vi "End.vi"(8 "error in (no error)":errorcluster, 11 "TelFocus in":refnum<class "TelFocus.lvclass">) -> (0 "error out":errorcluster, 3 "TelFocus out":refnum<class "TelFocus.lvclass">)   [LabVIEW 2018, in "TelFocus.lvclass"]
uses:
  TelFocus.lvclass
  Server/Server.lvclass
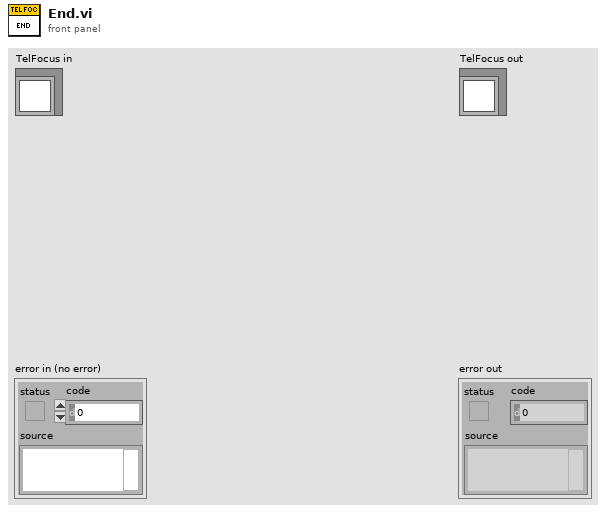
[diagram p1: front panel]
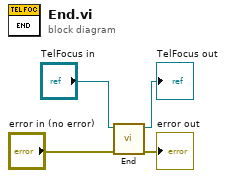
[diagram p0: block diagram]
diagram:
  n1 = call-parent "End.vi"("error in (no error)"="error in (no error)", "Server in"="TelFocus in") -> ("error out"=→"error out":errorcluster, "Server out"=→"TelFocus out":refnum<class "TelFocus.lvclass">)  [unwired: 8 in]
